vi "ADC_RangeAll.vi"(7 "DeviceIndex":u32, 8 "error in (no error)":errorcluster, 10 "bSingleEnded":bool=TRUE, 11 "pGainCodes":T1[](array[typedef])) -> (0 "error out":errorcluster)   [LabVIEW 2012]
uses:
  Controls/Gain Mode.ctl
  Windows/System32/AIOUSB.dll
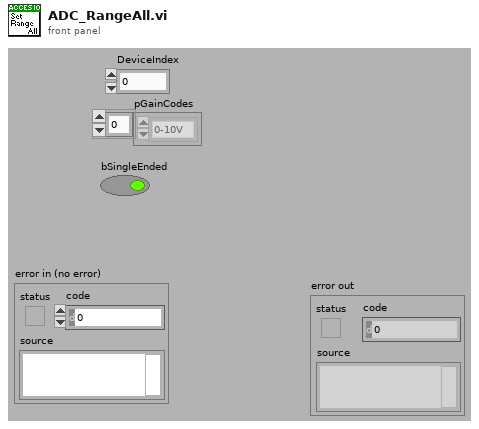
[diagram p1: front panel]
types:
  T1 = typedef "Gain Mode.ctl" = enum8{"0-10V", "+/- 10V", "0-5V", "+/- 5V", "0-2V", "+/- 2V", "0-1V", "+/- 1V"}
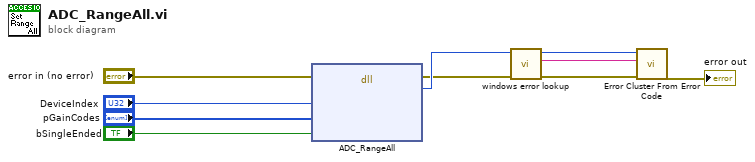
[diagram p0: block diagram]
diagram:
  n1 = dll-call lib="C:/Windows/System32/AIOUSB.dll" fn="ADC_RangeAll"(error in="error in (no error)", "DeviceIndex"="DeviceIndex", "pGainCodes"="pGainCodes", "bSingleEnded"="bSingleEnded") -> (error out=w3:errorcluster, "return type"=w4:u32)  [unwired: 5 in, 1 out]
  n2 = call "windows error lookup.vi"("error in (no error)"=w3, "Error Code"=w4) -> ("error out"=w2:errorcluster, "error message (\"\")"=w5:string)  [unwired: 8 in]
  n3 = call <vilib>:"Error Cluster From Error Code.vi"("error in (no error)"=w2, "error message (\"\")"=w5, "error code (0)"=w4) -> ("error out"=→"error out":errorcluster)  [unwired: 6 in]
